vi "Csv_read.vi"() -> ()   [LabVIEW 2016]
uses:
  <vilib>/Utility/file.llb/Read Delimited Spreadsheet (string).vi
panel:
  out "SR":dbl
  out "all rows 2":string[][](array[string])
  in  "file path (dialog if empty)":path
  out "Waveform Graph":waveform(dbl)[](graph)
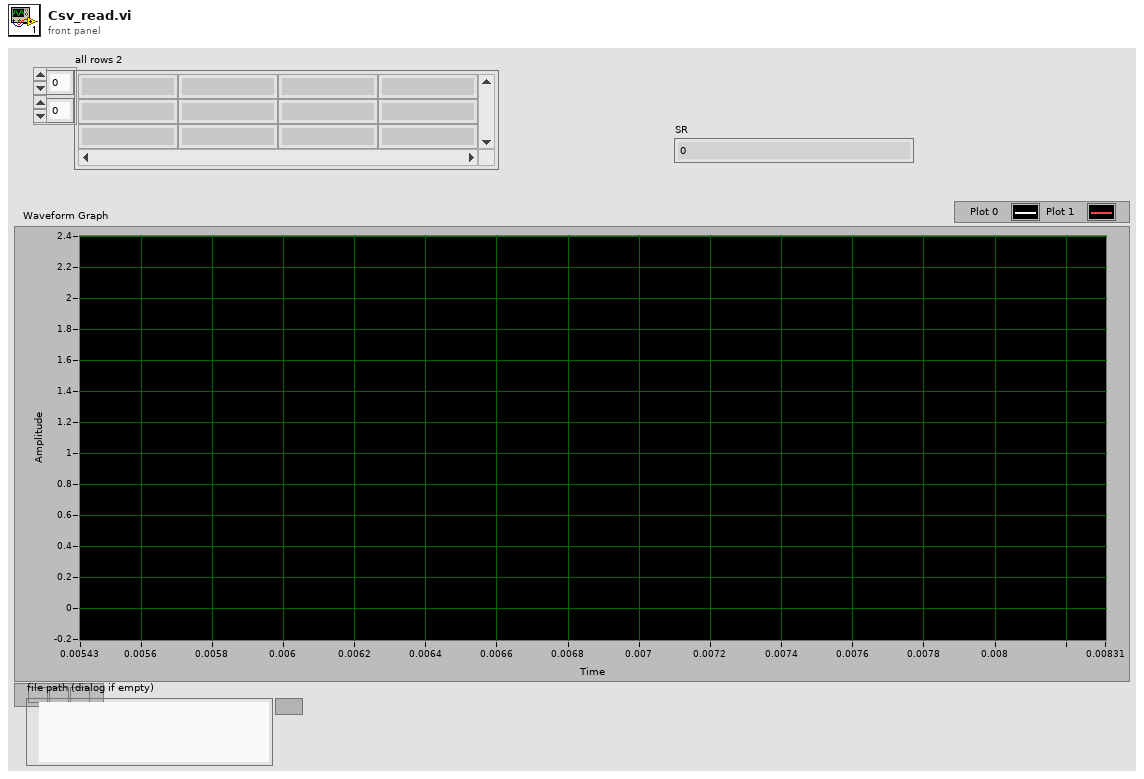
[diagram p1: front panel]
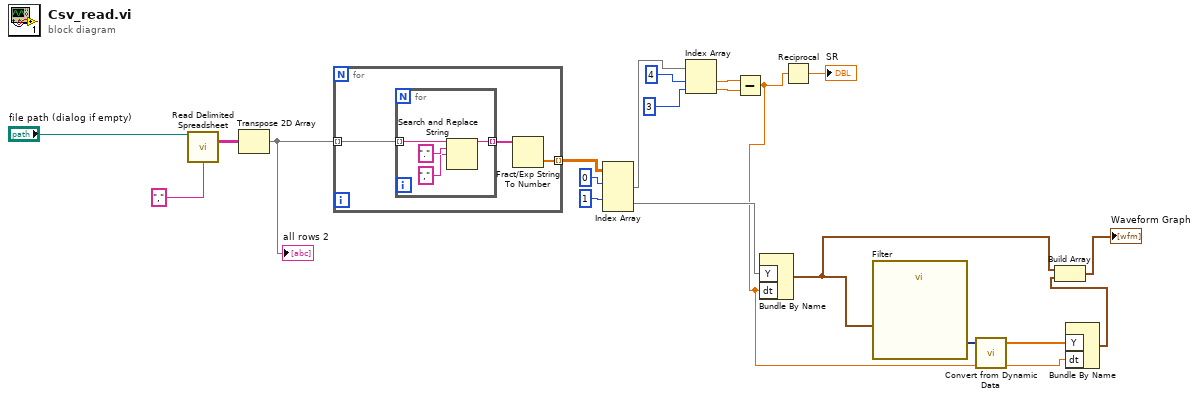
[diagram p0: block diagram]
diagram:
  n1 = call-poly <vilib>:"Read Delimited Spreadsheet.vi"("file path (dialog if empty)"="file path (dialog if empty)", "delimiter (\\t)"="," ("delimiter (\\t)")) -> ("all rows"=w18:string[][])  [unwired: 8 in, 5 out]
  n2 = Transpose 2D Array(2D array=w18) -> (transposed array=w15:string[][])
  "all rows 2" <- w15
  n3 = for {
    tunnel: [w23] -> w14 mode=indexing
    tunnel: w15 -> [w21] mode=indexing
    n4 = for {
      tunnel: w21 -> [w27] mode=indexing
      tunnel: [w24] -> w22 mode=indexing
      n5 = Search and Replace String(input string=w27, search string="." ("substring (\"\")"), replace string="," ("replace string (\"\")")) -> (result string=w24:string)  [unwired: 5 in, 3 out]
    }
    n6 = Fract/Exp String To Number(string=w22) -> (number=w23:dbl[])  [unwired: 3 in, 1 out]
  }
  n7 = Index Array(array=w14, index (row) #1=0 ("index (row)"), index (row) #2=1 ("index (row)")) -> (element #1=w12:dbl[], element #2=w13:dbl[])  [unwired: 2 in]
  n8 = Index Array(array=w12, index #1=4 ("index"), index #2=3 ("index")) -> (element #1=w8:dbl, element #2=w9:dbl)
  n9 = Subtract(x=w8, y=w9) -> (x-y=w3:dbl)
  n10 = Bundle By Name("Y"=w13, "dt"=w3) -> (w5:waveform(dbl))  [unwired: 1 in]
  n11 = Reciprocal(x=w3) -> (1/x=→"SR":dbl)
  n12 = call "Filter"("Signal"=w5) -> ("Filtered Signal"=w6:dynamicdata)  [unwired: 9 in, 1 out]
  n13 = call "Convert from Dynamic Data"("Dynamic Data Type"=w6) -> ("Array"=w4:dbl[])  [unwired: 3 in]
  n14 = Bundle By Name("Y"=w4, "dt"=w3) -> (w2:waveform(dbl))  [unwired: 1 in]
  n15 = Build Array(w5, w2) -> (→"Waveform Graph":waveform(dbl)[])
